vi "Check and Get Sizes.vi"(8 "error in (no error)":errorcluster, 9 "test commands":string[](array[string]), 10 "variable name":string, 11 "GOLPI ref. in":T1={"pipe handle"={"lv_proc.dll file path"=path "", "process instance handle"=[], "debug mode"=FALSE, "debug data"=[]}, "fast read timeout [ms]"=500, "fast read settle time [ms]"=10, "fast read to multiple [ms]"=1, "max elements per input line"=100, "slow read timeout [ms]"=5000, "stdin double format specifier"="%_16e", "max elements per stdout output column"=100, "console mode bitstream"=FALSE, "bitstream first read timeout [ms]"=1000, "bitstream read timeout [ms]"=50, "struct transfer possible"=FALSE, "matlab mode"=FALSE}) -> (0 "error out":errorcluster, 1 "octave sizes":i32[](array[numeric]), 2 "all tests OK?":bool, 3 "GOLPI ref. out":T1={"pipe handle"={"lv_proc.dll file path"=path "", "process instance handle"=[], "debug mode"=FALSE, "debug data"=[]}, "fast read timeout [ms]"=500, "fast read settle time [ms]"=10, "fast read to multiple [ms]"=1, "max elements per input line"=100, "slow read timeout [ms]"=5000, "stdin double format specifier"="%_16e", "max elements per stdout output column"=100, "console mode bitstream"=FALSE, "bitstream first read timeout [ms]"=1000, "bitstream read timeout [ms]"=50, "struct transfer possible"=FALSE, "matlab mode"=FALSE})   [LabVIEW 2020, in "GOLPI library.lvlib"]
doc: "Checks GNU Octave variable and gets its size. 'variable name' is the name of the variable. 'test commands' is array of GNU Octave commands with boolean output applied to the variable. I.e. to read noncomplex double scalar variable 'x', following array should be supplied:\nisnumeric\nisscalar\n~isscomplex\nTests performed are:\nisnumeric(x)\nisscalar(x)\n~iscomplex(x)\nIf output of all tests is '1', output 'all tests OK?' is true.\nReturns size of variable in GNU Octave metric (i.e. no elements with zero indexes)"
uses:
  GOLPI library.lvlib
  GOLPI reference Type Def.ctl
  Pipe Handle.ctl
  Custom Error Codes Enum Type Def.vi
  <vilib>/regexp/Match Regular Expression.xnode
  LV Process library.lvlib
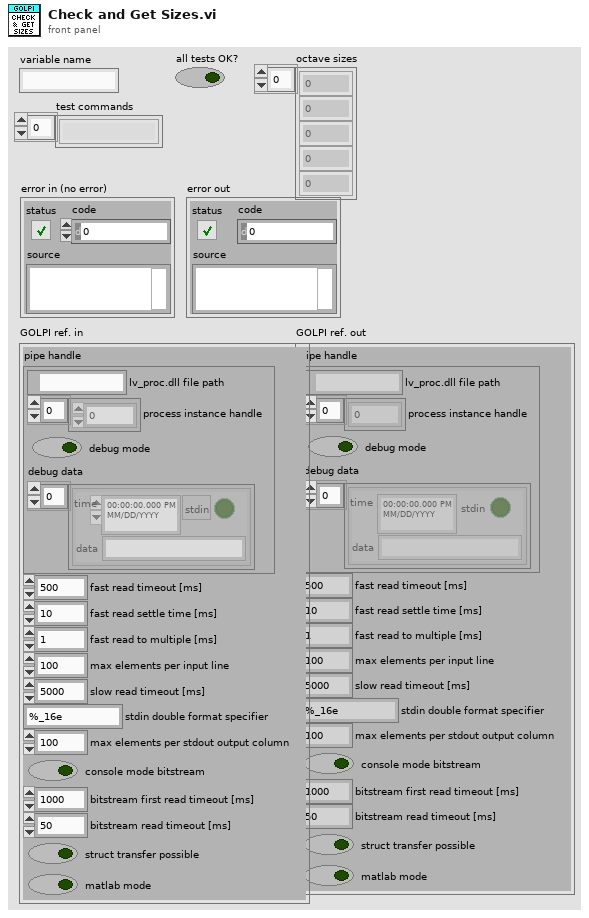
[diagram p1: front panel]
types:
  T1 = typedef "GOLPI library.lvlib/GOLPI reference Type Def.ctl" = cluster{"pipe handle":T2, "fast read timeout [ms]":u32, "fast read settle time [ms]":u32, "fast read to multiple [ms]":u32, "max elements per input line":u32, "slow read timeout [ms]":u32, "stdin double format specifier":string, "max elements per stdout output column":u32, "console mode bitstream":bool, "bitstream first read timeout [ms]":u32, "bitstream read timeout [ms]":u32, "struct transfer possible":bool, "matlab mode":bool}
  T2 = typedef "LV Process library.lvlib/Pipe Handle.ctl" = cluster{"lv_proc.dll file path":path, "process instance handle":u32[], "debug mode":bool, "debug data":cluster{"time":timestamp, "stdin":bool, "data":string}[]}
  T3 = typedef "GOLPI library.lvlib/Custom Error Codes Enum Type Def.vi" = enum16{"no error", "00 working directory PAR1 missing", "01 octave binary PAR1 missing", "02 octave report error PAR1", "03 empty output last cmd PAR1", "04 missing temporary file PAR1", "05 pwd PAR 1 not exist", "06 oct package not installed", "07 octave default binary missing", "10 var PAR1 not string, vect", "11 var PAR1 not num, scal, ~compl", "12 var PAR1 not num, scal, compl", "13 var PAR1 not num, vect, ~compl", "14 var PAR1 not num, vect, compl", "15 var PAR1 not num, mat, ~compl", "16 var PAR1 not num, mat, ~compl", "30 read timeout", "60 bitstream transport failed", "61 bitstream decode error PAR1", "62 bitstream cannot be set", "70 struct transfer not possible", "80 struct: cluster elem. PAR1 not implem.", "81 struct: structure field PAR1 not implem.", "82 struct: size mismatch of PAR1", "83 struct: type mismatch of PAR1", "98 internal error", "99 not finished", "90 Not supported in Matlab mode", "91 Matlab variable transfer error", "92 Matlab Script Error"}
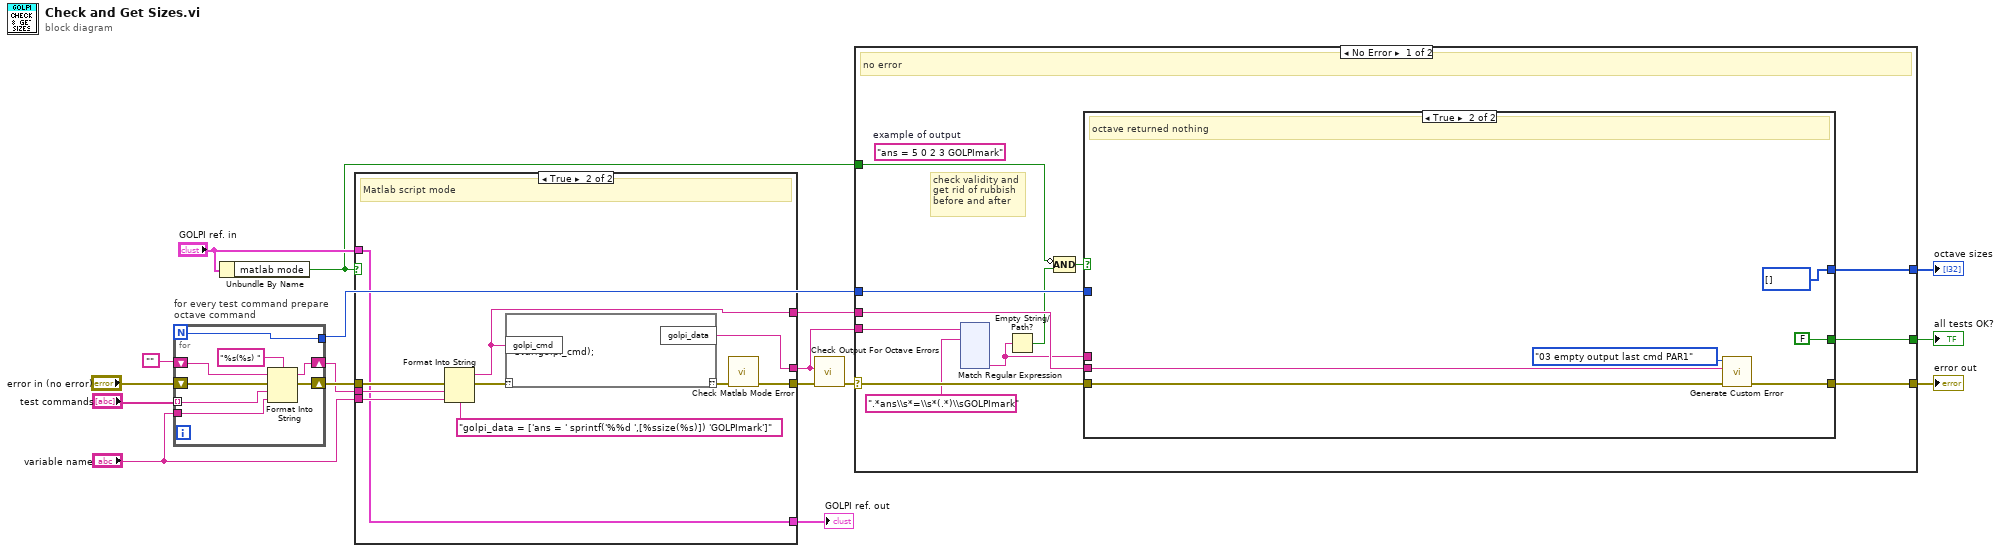
[diagram p0: block diagram]
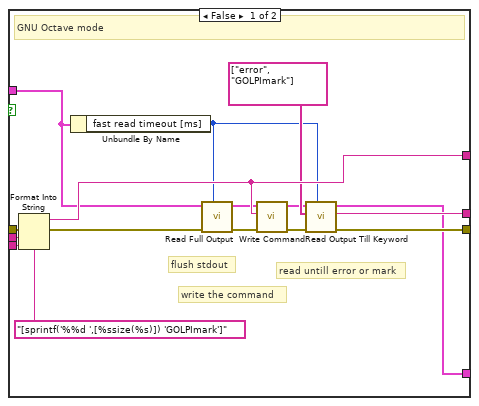
[diagram p2: hidden frame]
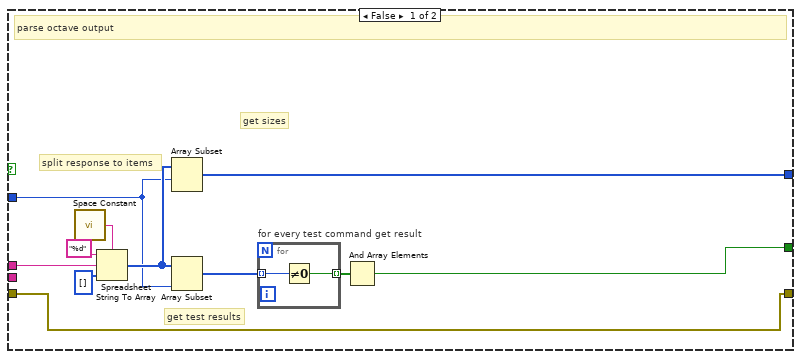
[diagram p3: hidden frame]
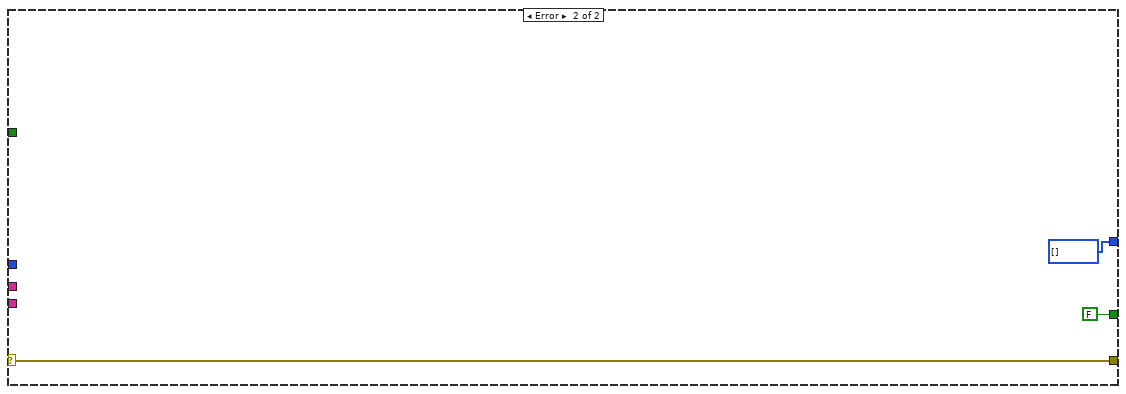
[diagram p4: hidden frame]
diagram:
  n1 = for "for every test command prepare\noctave command" {
    N -> [w18]
    tunnel: "test commands" -> [w23] mode=indexing
    tunnel: "variable name" -> [w22]
    shift-right: [w21] -> w4
    shift-left: "" -> [w24]
    shift-right: [w19] -> w5
    shift-left: "error in (no error)" -> [w20]
    tunnel: [w18] -> w8
    n2 = Format Into String(format string="%s(%s) ", initial string=w24, error in=w20, w23, w22) -> (resulting string=w21:string, error out=w19:errorcluster)
  }
  n3 = Unbundle By Name("GOLPI ref. in") -> ("matlab mode"=w2:bool)
  n4 = case shown="True" w2 {
    tunnel: [w41 w42] -> w13
    tunnel: [w40 w46] -> w12
    tunnel: [w39 w45] -> w9
    tunnel: "variable name" -> [w38 w48]
    tunnel: "GOLPI ref. in" -> [w37 w44]
    tunnel: w5 -> [w35 w51]
    tunnel: w4 -> [w27 w49]
    tunnel: [w26 w44] -> w1
    frame False {
      # "read untill error or mark"
      # "write the command"
      # "flush stdout"
      # "GNU Octave mode"
      n5 = Format Into String(format string="[sprintf('%%d ',[%ssize(%s)]) 'GOLPImark']", error in=w35, w27, w38) -> (resulting string=w39:string, error out=w34:errorcluster)  [unwired: 1 in]
      n6 = Unbundle By Name(w37) -> ("fast read timeout [ms]"=w28:u32)
      n7 = call "Read Full Output.vi"("timeout [ms]"=w28, "error in"=w34, "GOLPI ref. in"=w37) -> ("error out"=w33:errorcluster, "GOLPI ref. out"=w32:T1)  [unwired: 5 in, 2 out]
      n8 = call "Write Command.vi"("error in"=w33, "command"=w39, "GOLPI ref. in"=w32) -> ("error out"=w29:errorcluster, "GOLPI ref. out"=w30:T1)  [unwired: 7 in]
      n9 = call "Read Output Till Keyword.vi"("timeout [ms]"=w28, "error in"=w29, "keywords"=string[] ["error", "GOLPImark"], "GOLPI ref. in"=w30) -> ("error out"=w41:errorcluster, "read buffer"=w40:string, "GOLPI ref. out"=w26:T1)  [unwired: 4 in, 1 out]
    }
    frame True {
      # "Matlab script mode"
      n10 = Format Into String(format string="golpi_data = ['ans = ' sprintf('%%d ',[%ssize(%s)]) 'GOLPImark']", error in=w51, w49, w48) -> (resulting string=w45:string, error out=w47:errorcluster)  [unwired: 1 in]
      n11 = script code="eval(golpi_cmd);"("??"=w47, "golpi_cmd"=w45) -> ("??"=w43:errorcluster, "golpi_data"=w46:string)
      n12 = call "Check Matlab Mode Error.vi"("error in"=w43) -> ("error out"=w42:errorcluster)  [unwired: 10 in]
    }
  }
  "GOLPI ref. out" <- w1
  n13 = call "Check Output For Octave Errors.vi"("error in"=w13, "read buffer"=w12) -> ("error out"=w11:errorcluster)  [unwired: 9 in]
  n14 = case shown="No Error" w11 {
    selector: w11 -> [w61 w199]
    tunnel: [w63 FALSE] -> w15
    tunnel: [w62 i32[] []] -> w14
    tunnel: w12 -> [w56 _]
    tunnel: [w60 w199] -> w10
    tunnel: w9 -> [w59 _]
    tunnel: w8 -> [w58 _]
    tunnel: w2 -> [w52 _]
    frame No Error {
      (unwired) "ans = 5 0 2 3 GOLPImark"  # example of output
      # "check validity and\nget rid of rubbish\nbefore and after"
      # "no error"
      n15 = xnode "Match Regular Expression"("input string"=w56, "regular expression"=".*ans\\s*=\\s*(.*)\\sGOLPImark") -> ("submatch 1"=w57:string)  [unwired: 4 in, 5 out]
      n16 = Empty String/Path?(string/path=w57) -> (empty?=w53:bool)
      n17 = Compound Arithmetic op=AND(invert w52, w53) -> (w54:bool)
      n18 = case shown="True" w54 {
        tunnel: [w188 FALSE] -> w63
        tunnel: [w180 i32[] []] -> w62
        tunnel: w57 -> [w184 _]
        tunnel: w61 -> [w190 w195]
        tunnel: [w190 w194] -> w60
        tunnel: w59 -> [_ w193]
        tunnel: w58 -> [w181 _]
        frame False {
          # "get sizes"
          # "get test results"
          # "split response to items"
          # "parse octave output"
          n19 = call <vilib>:"Space Constant.vi"() -> ("String"=w185:string)
          n20 = Spreadsheet String To Array(delimiter (Tab)=w185, format string="%d", spreadsheet string=w184, array type (2D Dbl)=i32[] []) -> (array=w182:i32[])
          n21 = Array Subset(array=w182, index=w181) -> (w180:i32[])  [unwired: 1 in]
          n22 = Array Subset(array=w182, length=w181) -> (w183:i32[])  [unwired: 1 in]
          n23 = for "for every test command get result" {
            tunnel: w183 -> [w191] mode=indexing
            tunnel: [w192] -> w189 mode=indexing
            n24 = Not Equal To 0?(x=w191) -> (x != 0?=w192:bool)
          }
          n25 = And Array Elements(Boolean array=w189) -> (logical AND=w188:bool)
        }
        frame True {
          # "octave returned nothing"
          n26 = call "Generate Custom Error.vi"("error in"=w195, "PAR1"=w193, "GOLPI error"=Custom_Error_Codes_Enum_Type_Def.vi."03 empty output last cmd PAR1" ("Enum")) -> ("error out"=w194:errorcluster)  [unwired: 8 in]
        }
      }
    }
    frame Error {
    }
  }
  "all tests OK?" <- w15
  "octave sizes" <- w14
  "error out" <- w10
